vi "deg2ad.vi"(2 "DEC (°)":dbl format="%.8f", 3 "RA (°)":dbl format="%.8g") -> (0 "DEC (°)":dbl format="%<%H:%M:%S%1u>t", 1 "RA (sec)":dbl format="%<%H:%M:%S%2u>t")   [LabVIEW 2011]
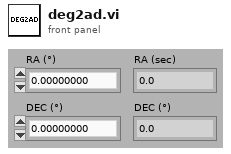
[diagram p1: front panel]
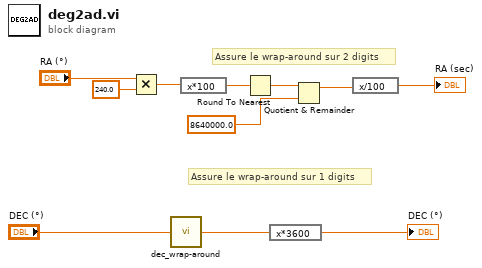
[diagram p0: block diagram]
diagram:
  # "Assure le wrap-around sur 1 digits"
  # "Assure le wrap-around sur 2 digits"
  n1 = Multiply(x="RA (°)", y=240.0) -> (x*y=w9:dbl)
  n2 = call "dec_wrap-around.vi"("DEC IN (°)"="DEC (°)") -> ("DEC OUT (°)"=w2:dbl)  [unwired: 14 in]
  n3 = expression code="x*100"(w9) -> (w8:dbl)
  n4 = Round To Nearest(number=w8) -> (nearest integer value=w6:dbl)
  n5 = expression code="x*3600"(w2) -> (→"DEC (°)":dbl)
  n6 = Quotient & Remainder(x=w6, y=8640000.0) -> (x-y*floor(x/y)=w5:dbl)  [unwired: 1 out]
  n7 = expression code="x/100"(w5) -> (→"RA (sec)":dbl)
